vi "CreateArbWfrm.vi"(8 "error in (no error)":errorcluster, 11 "ClassIn":refnum<class "Keysight335XX.lvclass">) -> (0 "error out":errorcluster, 3 "ClassOut":refnum<class "Keysight335XX.lvclass">)   [LabVIEW 2014, in "FGenPlugins.lvlib" / "Keysight335XX.lvclass"]
uses:
  Keysight335XX.lvclass
  <instrlib>/Agilent 3352X Series/Agilent 3352X Series.lvlib
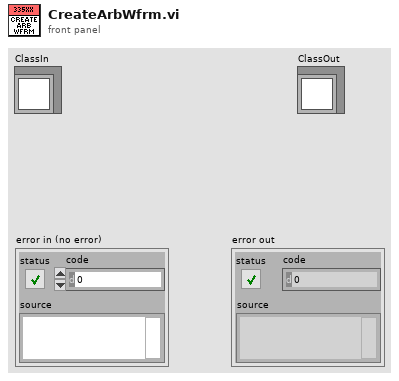
[diagram p1: front panel]
types:
  T1 = typedef "NISTFGenPlugins.lvlib/NISTFGenPluginsBase.lvclass/ArbWfrmParams.ctl" = cluster{"sWfrmHandle":string, "iSize":i32, "dData":dbl[], "dGain":dbl, "dOffset":dbl, "dSampleRate":dbl}
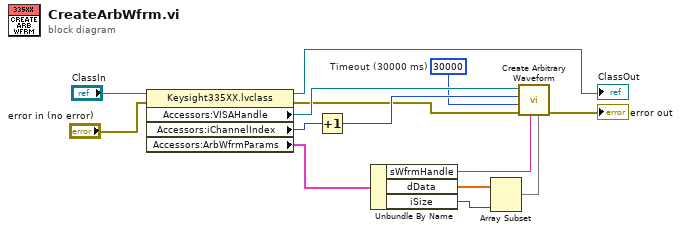
[diagram p0: block diagram]
diagram:
  w4 = u32 30000  # Timeout (30000 ms)
  n1 = property class="Keysight335XX.lvclass"(reference="ClassIn", error in="error in (no error)") -> (reference out=→"ClassOut":refnum<class "Keysight335XX.lvclass">, error out=w3:errorcluster, "Accessors:VISAHandle"=w12:refnum<visa-resource-name>, "Accessors:iChannelIndex"=w11:i32, "Accessors:ArbWfrmParams"=w9:T1)
  n2 = Increment(x=w11) -> (x+1=w10:i32)
  n3 = Unbundle By Name(w9) -> ("sWfrmHandle"=w8:string, "dData"=w7:dbl[], "iSize"=w6:i32)
  n4 = Array Subset(array=w7, length=w6) -> (w5:dbl[])  [unwired: 1 in]
  n5 = call <instrlib>:"Create Arbitrary Waveform.vi"("Arbitrary Waveform Data"=w5, "Arbitrary Waveform Name (ARB1)"=w8, "error in (no error)"=w3, "Timeout (10000 ms)"=w4, "Channel (1: 1)"=w10, "VISA resource name"=w12) -> ("error out"=→"error out":errorcluster)  [unwired: 1 in, 4 out]
